vi "GV_ZoomVerticalPerform.vi"(8 "error in (no error)":errorcluster, 9 "Coords":T1, 11 "Gviewer in":refnum<class "Gviewer.lvclass">) -> (0 "error out":errorcluster, 3 "Gviewer out":refnum<class "Gviewer.lvclass">)   [LabVIEW 2020, in "Gviewer.lvclass"]
doc: "Andre Koelewijn, 5 may 2021\n\nPerform the Vertical zoom action when the mouse button is released"
uses:
  Gviewer.lvclass
  <vilib>/Utility/miscctls.llb/LVPoint32TypeDef.ctl
  Gviewer.lvclass/Gviewer.ctl
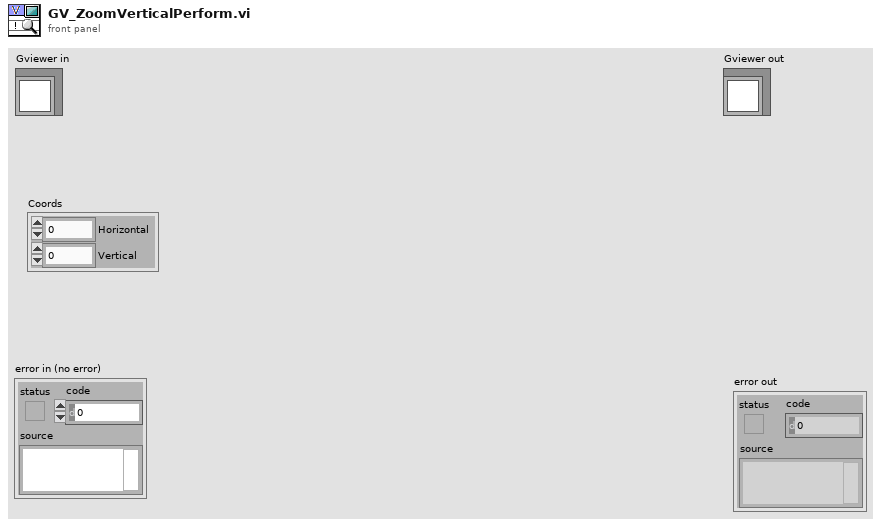
[diagram p1: front panel]
types:
  T1 = typedef "LVPoint32TypeDef.ctl" = cluster{"Horizontal":i32, "Vertical":i32}
  T2 = typedef "Gviewer.lvclass/Typedef_SelProperties.ctl" = cluster{"Color":u32, "LineType":T3, "max":dbl, "min":dbl}
  T3 = typedef "Gviewer.lvclass/Typedef_LineType.ctl" = enum16{"num_bare", "num_MinMax_Area", "num_MinMax_Lines", "num_MinMax_Forfor", "num_Max_Area", "num_Max_Line", "num_Max_Forfor", "num_Min_Area", "num_Min_Line", "num_Min_Fosfor", "Boolean_Line_01", "Boolean_Area_01", "Boolean_Fosfor_01", "Boolean_Line_TF", "Boolean_Area_TF", "Boolean_Fosfor_TF", "Boolean_OnOff_Line", "Boolean_OnOff_Area", "Boolean_OnOff_Fosfor", "Boolean_spare", "StringEvent_Line", "StringEvent_TimeLine"}
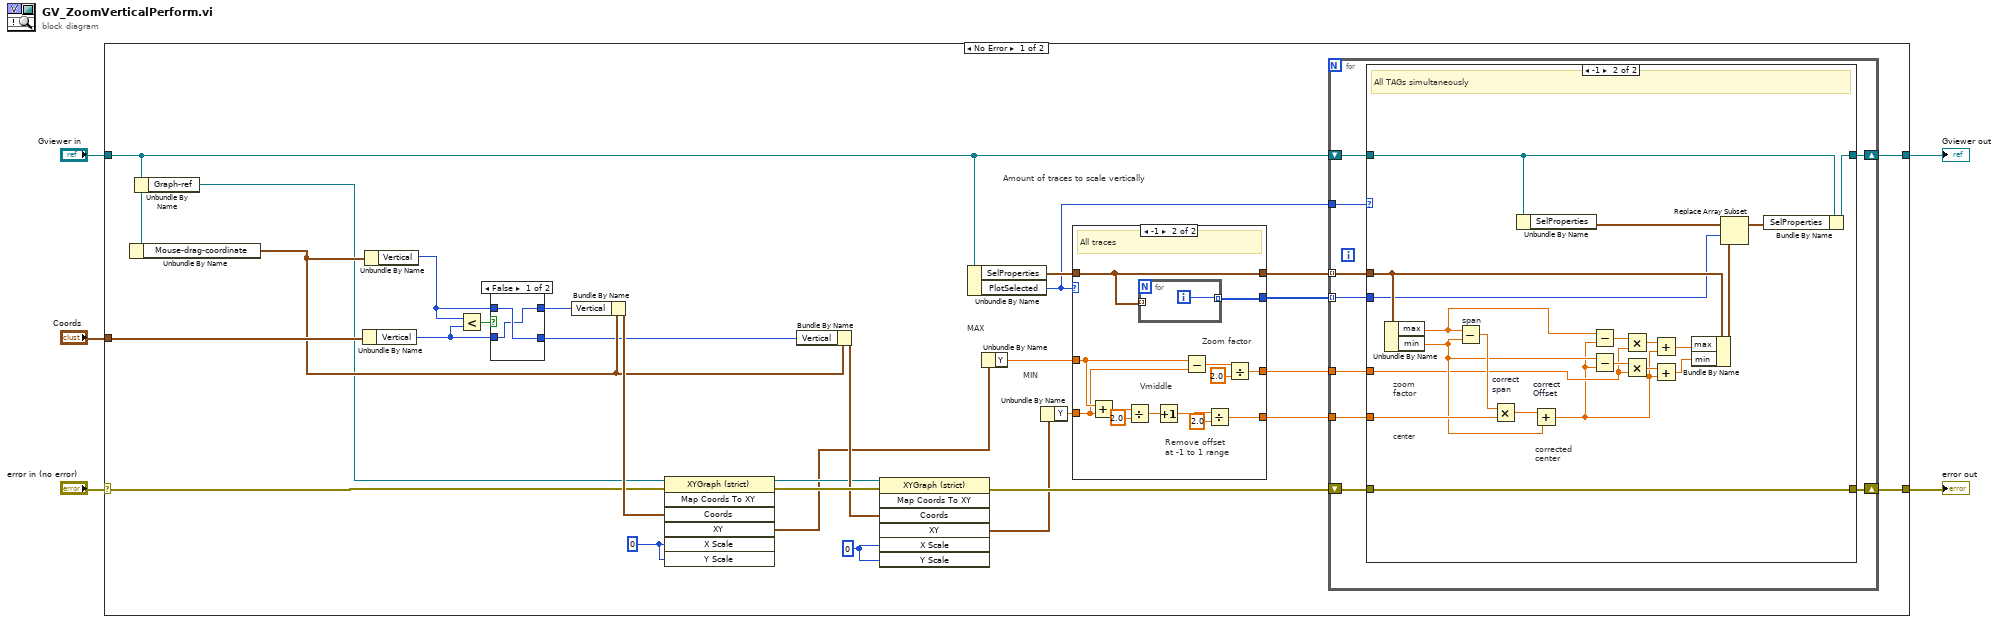
[diagram p0: block diagram]
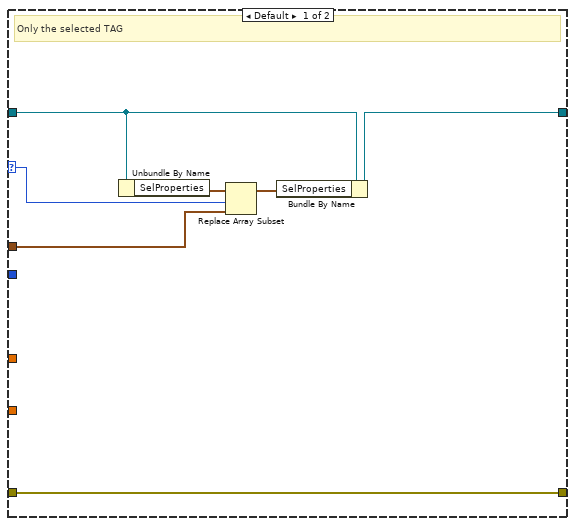
[diagram p2: hidden frame]
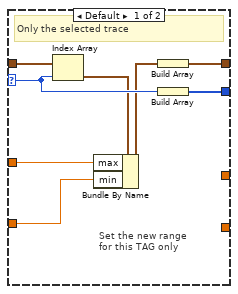
[diagram p3: hidden frame]
diagram:
  n1 = case shown="No Error" "error in (no error)" {
    selector: "error in (no error)" -> [w7 w99]
    tunnel: [w23 w99] -> w4
    tunnel: [w22 w98] -> w2
    tunnel: "Gviewer in" -> [w6 w98]
    tunnel: "Coords" -> [w27 _]
    frame No Error {
      w29 = 0 ("X Scale")
      w28 = 0 ("X Scale")
      # "MAX"
      # "MIN"
      # "Amount of traces to scale vertically"
      n2 = Unbundle By Name(w6) -> ("Mouse-drag-coordinate"=w21:T1)
      n3 = Unbundle By Name(w6) -> ("Graph-ref"=w8:refnum<vi>)
      n4 = Unbundle By Name(w27) -> ("Vertical"=w12:i32)
      n5 = Unbundle By Name(w21) -> ("Vertical"=w13:i32)
      n6 = Less?(x=w13, y=w12) -> (x < y?=w30:bool)
      n7 = case shown="False" w30 {
        tunnel: w13 -> [w95 w97]
        tunnel: [w94 w97] -> w14
        tunnel: [w95 w96] -> w15
        tunnel: w12 -> [w94 w96]
        frame False {
        }
        frame True {
        }
      }
      n8 = Bundle By Name(cluster=w21, "Vertical"=w14) -> (w31:T1)
      n9 = invoke class="XYGraph (strict)" method="Map Coords To XY"(reference=w8, error in=w7, "Coords"=w31, "X Scale"=w28, "Y Scale"=w28) -> (reference out=w32:refnum<vi>, error out=w34:errorcluster, "XY"=w17:cluster{"X":dbl, "Y":dbl})  [unwired: 2 in, 4 out]
      n10 = Bundle By Name(cluster=w21, "Vertical"=w15) -> (w33:T1)
      n11 = invoke class="XYGraph (strict)" method="Map Coords To XY"(reference=w32, error in=w34, "Coords"=w33, "X Scale"=w29, "Y Scale"=w29) -> (error out=w24:errorcluster, "XY"=w19:cluster{"X":dbl, "Y":dbl})  [unwired: 2 in, 5 out]
      n12 = Unbundle By Name(w6) -> ("SelProperties"=w26:T2[], "PlotSelected"=w9:i32)
      n13 = Unbundle By Name(w17) -> ("Y"=w16:dbl)
      n14 = Unbundle By Name(w19) -> ("Y"=w18:dbl)
      n15 = case shown="-1" w9 {
        selector: w9 -> [w77 _]
        tunnel: w26 -> [w78 w91]
        tunnel: [w79 w91] -> w20
        tunnel: [w76 w92] -> w25
        tunnel: w18 -> [w72 w83]
        tunnel: w16 -> [w73 w84]
        tunnel: [_ w85] -> w11
        tunnel: [_ w80] -> w10
        frame Default {
          # "Set the new range\nfor this TAG only"
          # "Only the selected trace"
          n16 = Index Array(array=w78, index=w77) -> (element=w75:T2)
          n17 = Bundle By Name(cluster=w75, "max"=w73, "min"=w72) -> (w74:T2)
          n18 = Build Array(w74) -> (w79:T2[])
          n19 = Build Array(w77) -> (w76:i32[])
        }
        frame -1 {
          # "Zoom factor"
          # "Remove offset\nat -1 to 1 range"
          # "Vmiddle"
          # "All traces"
          n20 = Add(x=w84, y=w83) -> (x+y=w90:dbl)
          n21 = Divide(x=w90, y=2.0) -> (x/y=w88:dbl)
          n22 = for {
            tunnel: [w93] -> w92 mode=indexing
            tunnel: w91 -> [_] mode=indexing
            i -> [w93]
          }
          n23 = Increment ("remove offset\nat -1 to 1 range")(x=w88) -> (x+1=w86:dbl)
          n24 = Subtract(x=w84, y=w83) -> (x-y=w81:dbl)
          n25 = Divide(x=w86, y=2.0) -> (x/y=w85:dbl)
          n26 = Divide(x=w81, y=2.0) -> (x/y=w80:dbl)
        }
      }
      n27 = for {
        tunnel: w20 -> [w41] mode=indexing
        tunnel: w25 -> [w36] mode=indexing
        shift-right: [w42] -> w22
        shift-left: w6 -> [w43]
        shift-right: [w39] -> w23
        shift-left: w24 -> [w40]
        tunnel: w11 -> [w38]
        tunnel: w10 -> [w37]
        tunnel: w9 -> [w35]
        n28 = case shown="-1" w35 {
          selector: w35 -> [w48 _]
          tunnel: w43 -> [w50 w69]
          tunnel: [w49 w68] -> w42
          tunnel: w41 -> [w47 w52]
          tunnel: w40 -> [w46 w67]
          tunnel: [w46 w67] -> w39
          tunnel: w38 -> [_ w66]
          tunnel: w37 -> [_ w59]
          tunnel: w36 -> [_ w51]
          frame Default {
            # "Only the selected TAG"
            n29 = Unbundle By Name(w50) -> ("SelProperties"=w44:T2[])
            n30 = Replace Array Subset(array=w44, new element=w47, index=w48) -> (w45:T2[])
            n31 = Bundle By Name(cluster=w50, "SelProperties"=w45) -> (w49:refnum<class "Gviewer.lvclass">)
          }
          frame -1 {
            # "corrected\ncenter"
            # "zoom\nfactor"
            # "center"
            # "All TAGs simultaneously"
            n32 = Unbundle By Name(w52) -> ("max"=w63:dbl, "min"=w62:dbl)
            n33 = Subtract "span"(x=w63, y=w62) -> (x-y=w65:dbl)
            n34 = Multiply "correct\nspan"(x=w65, y=w66) -> (x*y=w64:dbl)
            n35 = Unbundle By Name(w69) -> ("SelProperties"=w70:T2[])
            n36 = Add "correct\nOffset"(x=w64, y=w62) -> (x+y=w56:dbl)
            n37 = Subtract(x=w63, y=w56) -> (x-y=w60:dbl)
            n38 = Subtract(x=w62, y=w56) -> (x-y=w61:dbl)
            n39 = Multiply(x=w60, y=w59) -> (x*y=w58:dbl)
            n40 = Multiply(x=w61, y=w59) -> (x*y=w57:dbl)
            n41 = Add(x=w58, y=w56) -> (x+y=w55:dbl)
            n42 = Add(x=w57, y=w56) -> (x+y=w54:dbl)
            n43 = Bundle By Name(cluster=w52, "max"=w55, "min"=w54) -> (w53:T2)
            n44 = Replace Array Subset(array=w70, new element=w53, index=w51) -> (w71:T2[])
            n45 = Bundle By Name(cluster=w69, "SelProperties"=w71) -> (w68:refnum<class "Gviewer.lvclass">)
          }
        }
      }
    }
    frame Error {
    }
  }
  "error out" <- w4
  "Gviewer out" <- w2
